vi "Resource.vi"(8 "error in (no error)":errorcluster, 11 "Channel in":refnum<class "Channel.lvclass">) -> (0 "error out":errorcluster, 2 "Resource":string, 3 "Channel out":refnum<class "Channel.lvclass">)   [LabVIEW 2020, in "VolatusConfig.lvlib" / "Channel.lvclass"]
uses:
  Channel.lvclass
  Channel.lvclass/Channel.ctl
  lv-cdm/CDM-Config/Config Element/Config Element.lvclass
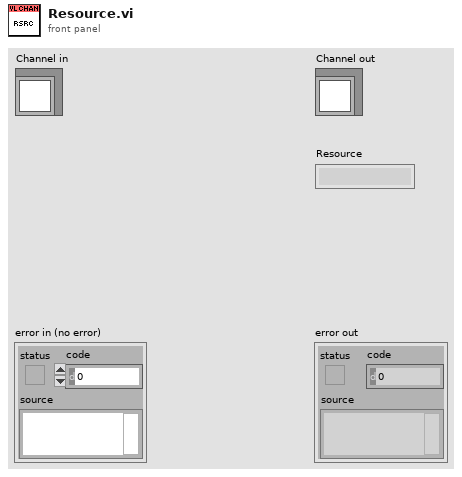
[diagram p1: front panel]
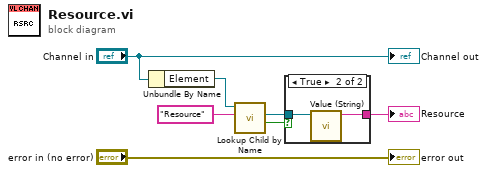
[diagram p0: block diagram]
diagram:
  n1 = Unbundle By Name("Channel in") -> ("Element"=w5:refnum<class "Config Element.lvclass">)
  n2 = call "Lookup Child by Name.vi"("Name"="Resource", "Config Element in"=w5) -> ("Found"=w3:bool, "Child"=w2:refnum<class "Config Element.lvclass">)  [unwired: 6 in, 2 out]
  n3 = case shown="True" w3 {
    tunnel: w2 -> [_ w9]
    tunnel: [_ w8] -> w1
    frame False {
    }
    frame True {
      n4 = call "Value (String).vi"("Config Element in"=w9) -> ("String Value"=w8:string)  [unwired: 9 in, 1 out]
    }
  }
  "Resource" <- w1
  "error out" <- "error in (no error)"
  "Channel out" <- "Channel in"
